vi "TreeInfor.vi"() -> (2 "Array":string[][](array[string])=[["Device", "Device", "0", "List.png"], ["PXI-6251", "PXI6251", "1", "Card.png"], ["Analog input", "ai", "2", "Channel.png"], ["PXI-6120", "PXI6120", "1", "Card.png"], ["Analog input", "Sai", "2", "DRP.png"], ["PXI-6704", "PXI6704", "1", "Card.png"], ["Analog output", "ao", "2", "Channel.png"], ["PXI-6514", "PXI651", "1", "Card.png"], ["Digital I/O", "dio", "2", "Channel.png"], ["PXI-8341", "PXI8341", "1", "Card.png"], ["RS 485", "com", "2", "Channel.png"]])   [LabVIEW 2017]
panel:
  in  "Tree":string[][](table)=[["Device", "Device", "0", "List.png"], ["PXI-6251", "PXI6251", "1", "Card.png"], ["Analog input", "ai", "2", "Channel.png"], ["PXI-6120", "PXI6120", "1", "Card.png"], ["Analog input", "Sai", "2", "DRP.png"], ["PXI-6704", "PXI6704", "1", "Card.png"], ["Analog output", "ao", "2", "Channel.png"], ["PXI-6514", "PXI6514", "1", "Card.png"], ["Digital I/O", "dio", "2", "Channel.png"], ["PXI-8431_6slot", "PXI8431_6", "1", "Card.png"], ["RS 422", "com_slot6", "2", "Channel.png"], ["PXI-8431_7slot", "PXI8431_7", "1", "Card.png"], ["RS 422", "com_slot7", "2", "Channel.png"], ["TDMS View", "TDMSview", "0", "Data,png"]]
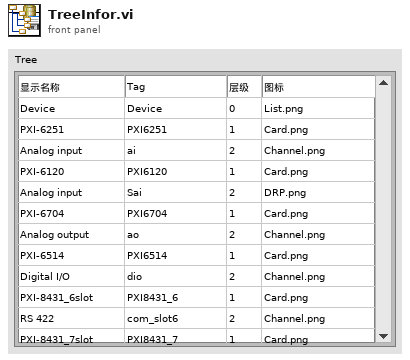
[diagram p1: front panel]
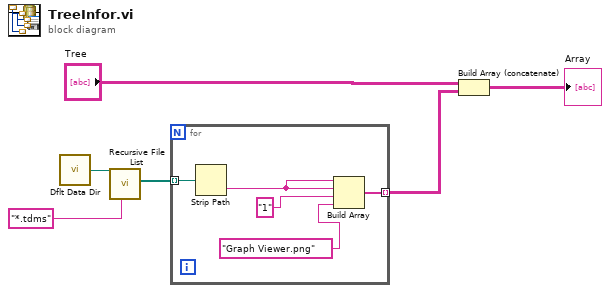
[diagram p0: block diagram]
diagram:
  n1 = call <vilib>:"Dflt Data Dir.vi"() -> ("App:Default Data Directory"=w4:path)
  n2 = call <vilib>:"Recursive File List.vi"("pattern"="*.tdms", "Folder Path"=w4) -> ("All Files in Dir"=w2:path[])  [unwired: 5 in, 4 out]
  n3 = for {
    tunnel: w2 -> [w11] mode=indexing
    tunnel: [w7] -> w1 mode=indexing
    n4 = Strip Path(path=w11) -> (name=w10:string)  [unwired: 1 out]
    n5 = Build Array(w10, w10, "1", "Graph Viewer.png") -> (w7:string[])
  }
  n6 = Build Array (concatenate)("Tree", w1) -> (→"Array":string[][])
